vi "Datasheet Check Logo West.vi"(5 "Company_ID_Txt":string) -> (0 "Insertion Height":string, 1 "Insertion Width":string, 2 "Company_ID_Txt":string)   [LabVIEW 2011]
uses:
  Summitek EXT/OpenG EXT/file/file.llb/File Exists - Scalar__ogtk.vi
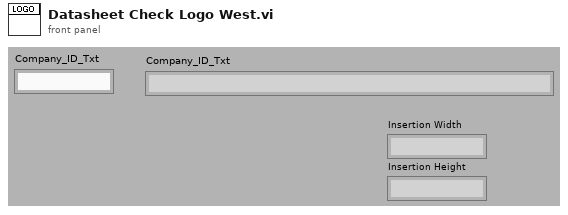
[diagram p1: front panel]
types:
  T1 = typedef "imagedata.ctl" = cluster{"image type":i32, "image depth":i32, "image":u8[], "mask":u8[], "colors":u32[], "Rectangle":cluster{"left":i16, "top":i16, "right":i16, "bottom":i16}}
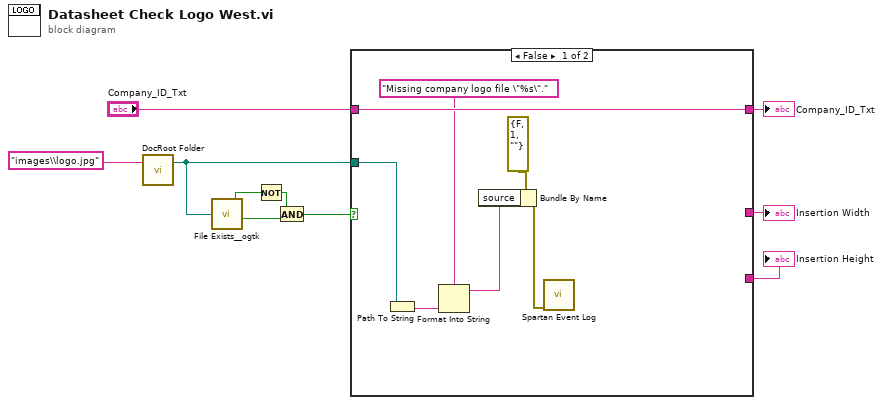
[diagram p0: block diagram]
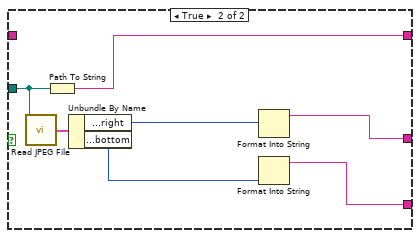
[diagram p2: hidden frame]
diagram:
  n1 = call "DocRoot Folder.vi"("Relative Path (\"\" - Folder)"="images\\logo.jpg") -> ("DocumentRoot Folder"=w1:path)  [unwired: 2 in]
  n2 = call-poly "File Exists__ogtk.vi"("file path"=w1) -> ("is directory"=w7:bool, "exists"=w8:bool)  [unwired: 6 in]
  n3 = Not(x=w7) -> (.not. x?=w6:bool)
  n4 = And(x=w6, y=w8) -> (x .and. y?=w5:bool)
  n5 = case shown="False" w5 {
    tunnel: "Company_ID_Txt" -> [w17 _]
    tunnel: [w17 w23] -> w9
    tunnel: w1 -> [w12 w24]
    tunnel: [_ w21] -> w4
    tunnel: [_ w20] -> w3
    frame False {
      n6 = Path To String(path=w12) -> (string=w11:string)
      n7 = Format Into String(format string="Missing company logo file \"%s\"." ("source"), w11) -> (resulting string=w13:string)  [unwired: 2 in, 1 out]
      n8 = Bundle By Name(cluster=errorcluster {"status"=FALSE, "code"=1, "source"=""} ("error in (no error)"), "source"=w13) -> (w15:errorcluster)
      n9 = call "Spartan Event Log.vi"("error in (no error)"=w15) -> ()  [unwired: 7 in, 1 out]
    }
    frame True {
      n10 = call <vilib>:"Read JPEG File.vi"("path to JPEG file"=w24) -> ("image data"=w22:T1)  [unwired: 1 in, 9 out]
      n11 = Path To String(path=w24) -> (string=w23:string)
      n12 = Unbundle By Name(w22) -> ("Rectangle.right"=w19:i16, "Rectangle.bottom"=w18:i16)
      n13 = Format Into String(w19) -> (resulting string=w21:string)  [unwired: 3 in, 1 out]
      n14 = Format Into String(w18) -> (resulting string=w20:string)  [unwired: 3 in, 1 out]
    }
  }
  "Company_ID_Txt" <- w9
  "Insertion Width" <- w4
  "Insertion Height" <- w3
